vi "update tree control.vi"(8 "error in":errorcluster, 10 "tree reference":refnum<vi>, 11 "glyph manager in":T1) -> (0 "error out":errorcluster, 3 "glyph manager out":T1)   [LabVIEW 2025, in "CEF.lvlib"]
doc: "Copyright 2017 National Instruments Corporation\n\nLicensed under the Apache License, Version 2.0 (the \"License\"); you may not use this file except in compliance with the License. You may obtain a copy of the License at http://www.apache.org/licenses/LICENSE-2.0\nUnless required by applicable law or agreed to in writing, software distributed under the License is distributed on an \"AS IS\" BASIS, WITHOUT WARRANTIES OR CONDITIONS OF ANY KIND, either express or implied. See the License for the specific language governing permissions and limitations under the License."
uses:
  CEF.lvlib
  glyph manager.ctl
  <vilib>/picture/picture.llb/imagedata.ctl
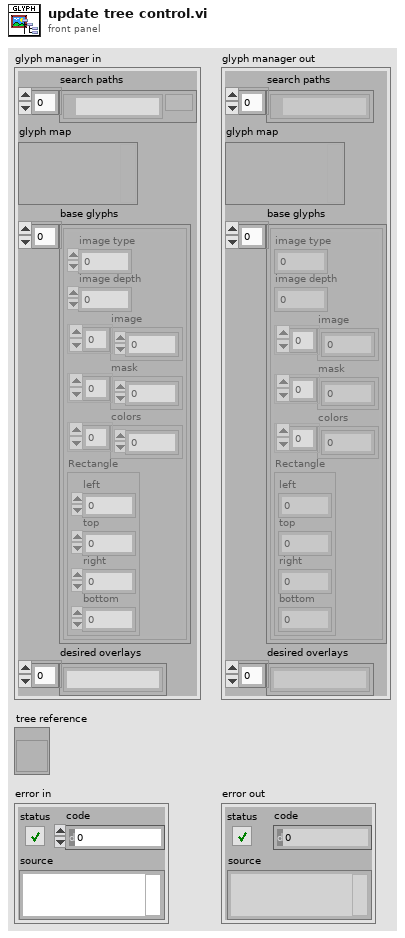
[diagram p1: front panel]
types:
  T1 = typedef "CEF.lvlib/glyph manager.ctl" = cluster{"search paths":path[], "glyph map":variant, "base glyphs":T2[], "desired overlays":string[]}
  T2 = typedef "imagedata.ctl" = cluster{"image type":i32, "image depth":i32, "image":u8[], "mask":u8[], "colors":u32[], "Rectangle":cluster{"left":i16, "top":i16, "right":i16, "bottom":i16}}
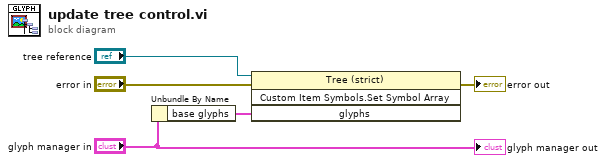
[diagram p0: block diagram]
diagram:
  n1 = Unbundle By Name("glyph manager in") -> ("base glyphs"=w2:T2[])
  n2 = invoke class="Tree (strict)" method="Custom Item Symbols.Set Symbol Array"(reference="tree reference", error in="error in", "glyphs"=w2) -> (error out=→"error out":errorcluster)  [unwired: 1 in, 3 out]
  "glyph manager out" <- "glyph manager in"
